vi "Variant To String.vi"(4 "Type Enum [auto]":T1, 5 "Formatting (auto)":string, 6 "Variant Type\\default":variant, 7 "Name (error)":string, 8 "error in (no error)":errorcluster, 10 "Multiply":variant, 11 "Registry Object":refnum<class "Carya Config.lvclass">) -> (0 "error out":errorcluster, 2 "String":string, 3 "Registry Object":refnum<class "Carya Config.lvclass">)   [LabVIEW 2013, in "Carya Config.lvclass"]
doc: "Copyright 2018, Carya Automatisering, Wiebe Walstra."
uses:
  Carya Config.lvclass
  <vilib>/Utility/VariantDataType/Type.ctl
  <vilib>/Utility/error.llb/Error Cluster From Error Code.vi
  <vilib>/regexp/Match Regular Expression.xnode
  <vilib>/ErrorRing/Error Ring.xnode
  <vilib>/Utility/VariantDataType/VariantType.lvlib
  CConfig Variant Accessor/CConfig Variant Accessor.lvclass
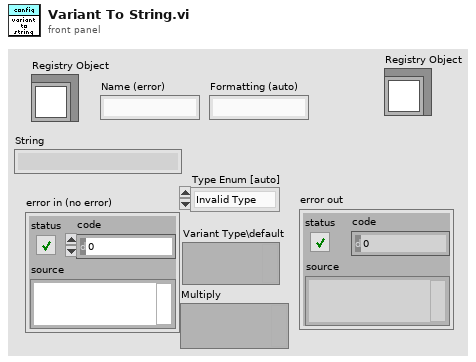
[diagram p1: front panel]
types:
  T1 = typedef "VariantType.lvlib/Type.ctl" = enum8{"Invalid Type", "Void", "I8", "I16", "I32", "I64", "U8", "U16", "U32", "U64", "Single Float", "Double Float", "Extended Float", "Single Complex", "Double Complex", "Extended Complex", "Enum U8", "Enum U16", "Enum U32", "Enum U64", "Single Float With Unit", "Double Float With Unit", "Extended Float With Unit", "Single Complex with Unit", "Double Complex with Unit", "Extended Complex with Unit", "Boolean", "String", "Path", "Picture", "Tag", "Array", "Cluster", "Variant", "LV Variant", "Waveform", "Timestamp", "Digital Waveform", "Digital Data", "ExpressData", "Refnum", "External Data", "VI", "Poly VI", "LabVIEW Class Instance", "Fixed Point"}
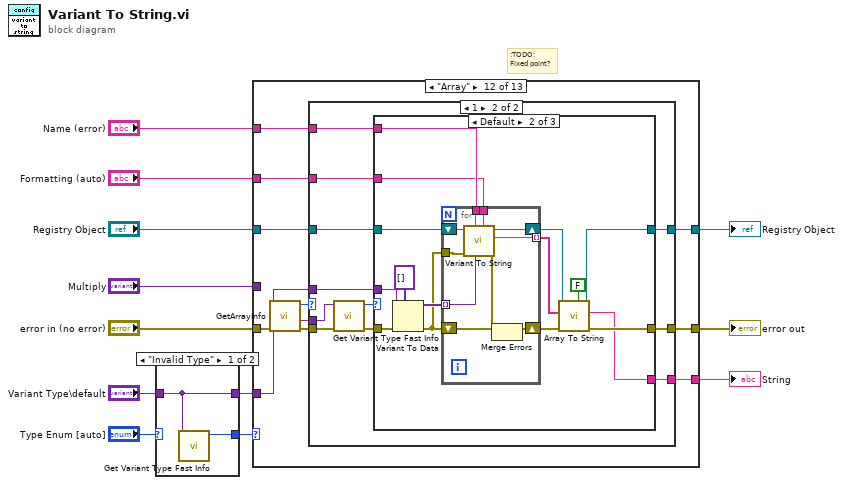
[diagram p0: block diagram]
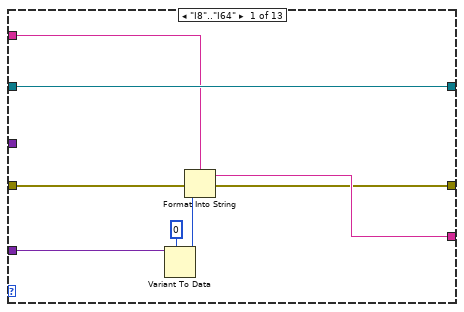
[diagram p2: hidden frame]
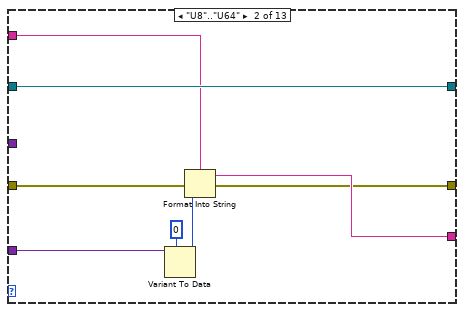
[diagram p3: hidden frame]
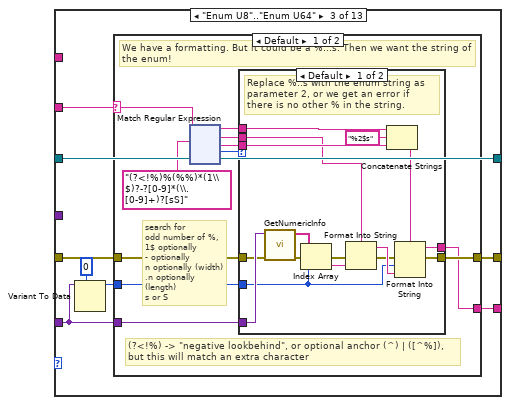
[diagram p4: hidden frame]
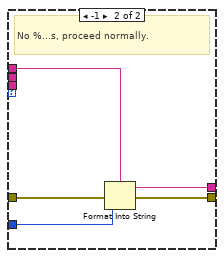
[diagram p5: hidden frame]
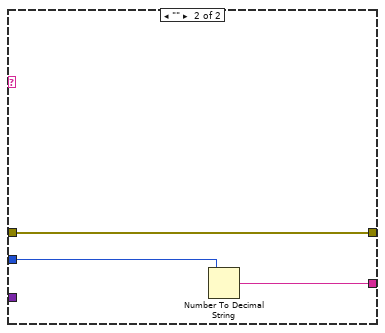
[diagram p6: hidden frame]
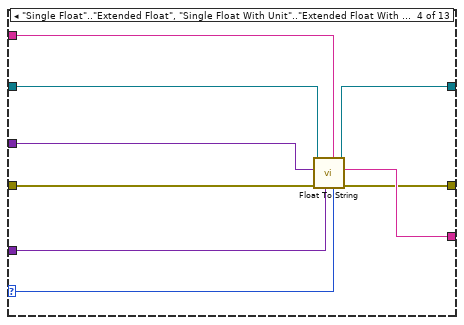
[diagram p7: hidden frame]
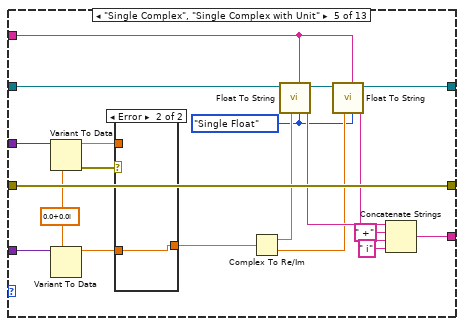
[diagram p8: hidden frame]
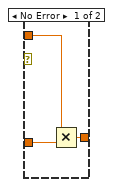
[diagram p9: hidden frame]
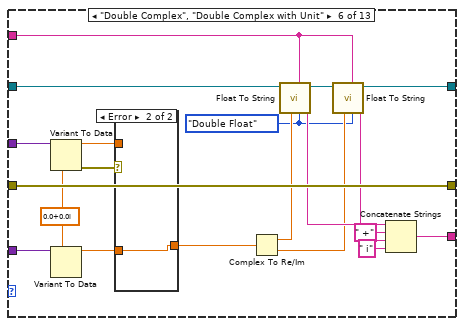
[diagram p10: hidden frame]
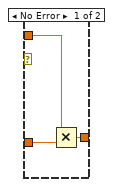
[diagram p11: hidden frame]
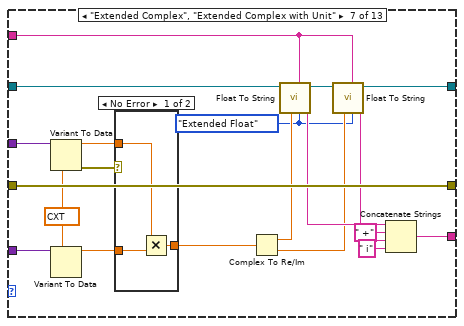
[diagram p12: hidden frame]
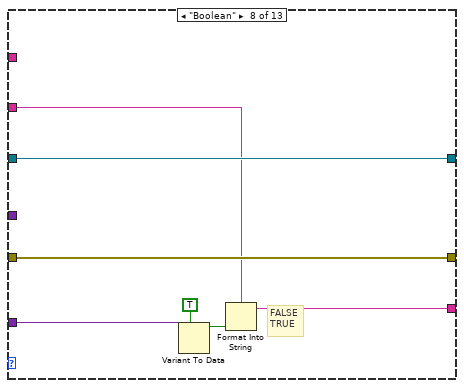
[diagram p14: hidden frame]
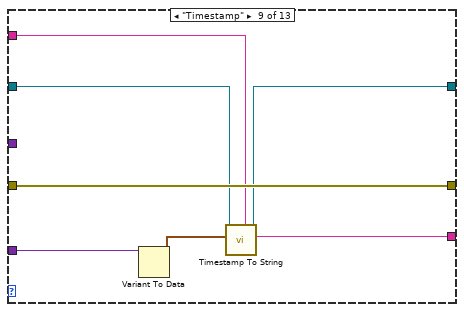
[diagram p15: hidden frame]
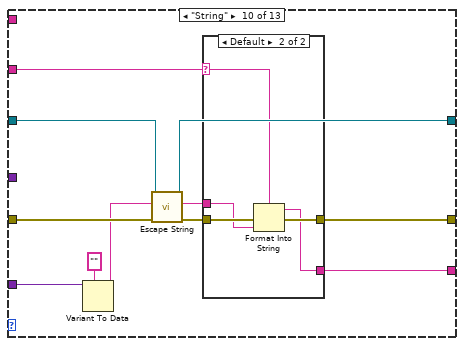
[diagram p16: hidden frame]
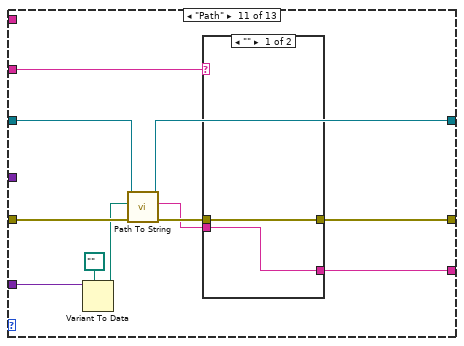
[diagram p18: hidden frame]
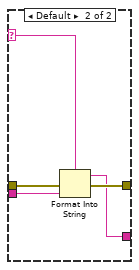
[diagram p19: hidden frame]
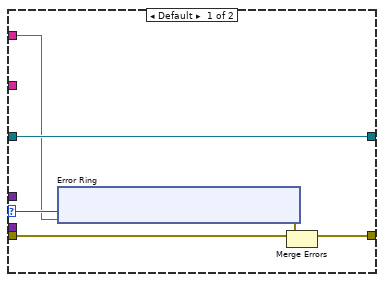
[diagram p20: hidden frame]
diagram:
  # ":TODO:\nFixed point?"
  n1 = case shown="\"Invalid Type\"" "Type Enum [auto]" {
    selector: "Type Enum [auto]" -> [_ w16]
    tunnel: "Variant Type\\default" -> [w13 w15]
    tunnel: [w14 w16] -> w7
    tunnel: [w13 w15] -> w8
    frame "Invalid Type" {
      n2 = call "Get Variant Type Fast Info.vi"("Variant"=w13) -> ("Type Enum"=w14:T1)  [unwired: 6 in, 4 out]
    }
    frame Default {
    }
  }
  n3 = case shown="\"Array\"" w7 {
    selector: w7 -> [_ _ _ w190 _ _ _ _ _ _ _ _ w409]
    tunnel: [w17 w25 w36 w191 w217 w241 w265 w274 w282 w287 w306 w328 w411] -> w10
    tunnel: "error in (no error)" -> [w18 w26 w37 w193 w217 w241 w265 w274 w282 w293 w311 w322 w413]
    tunnel: "Registry Object" -> [w20 w29 w40 w194 w204 w228 w252 w273 w281 w291 w309 w330 w412]
    tunnel: [w20 w29 w40 w197 w215 w239 w263 w273 w280 w290 w308 w329 w412] -> w4
    tunnel: w8 -> [w24 w32 w34 w192 w206 w230 w254 w276 w283 w294 w312 w327 _]
    tunnel: [w21 w28 w39 w196 w210 w234 w258 w271 w277 w285 w304 w325 _] -> w6
    tunnel: "Name (error)" -> [_ _ _ _ _ _ _ _ _ _ _ w324 w406]
    tunnel: "Formatting (auto)" -> [w19 w27 w38 w195 w209 w233 w257 w270 w278 w284 w303 w320 _]
    tunnel: "Multiply" -> [_ _ _ w189 w203 w227 w251 _ _ _ _ _ _]
    frame "I8".."I64" {
      n4 = Variant To Data(type=i64 0, Variant=w24) -> (data=w22:i64)  [unwired: 1 in, 1 out]
      n5 = Format Into String(format string=w19, error in=w18, w22) -> (resulting string=w21:string, error out=w17:errorcluster)  [unwired: 1 in]
    }
    frame "U8".."U64" {
      n6 = Variant To Data(type=u64 0, Variant=w32) -> (data=w30:u64)  [unwired: 1 in, 1 out]
      n7 = Format Into String(format string=w27, error in=w26, w30) -> (resulting string=w28:string, error out=w25:errorcluster)  [unwired: 1 in]
    }
    frame "Enum U8".."Enum U64" {
      n8 = Variant To Data(type=u64 0 ("unsigned 64bit integer"), Variant=w34) -> (data=w33:u64)  [unwired: 1 in, 1 out]
      n9 = case shown="Default" w38 {
        selector: w38 -> [w46 _]
        tunnel: w34 -> [w45 _]
        tunnel: [w42 w188] -> w39
        tunnel: w37 -> [w44 w186]
        tunnel: [w43 w186] -> w36
        tunnel: w33 -> [w41 w187]
        frame Default {
          # "(?<!%) -> \"negative lookbehind\", or optional anchor (^) | ([^%]), but this will match an extra character"
          # "search for\nodd number of %,\n1$ optionally\n- optionally\nn optionally (width)\n.n optionally (length)\ns or S"
          # "We have a formatting. But it could be a %...s. Then we want the string of the enum!"
          n10 = xnode "Match Regular Expression"("input string"=w46, "regular expression"="(?<!%)%(%%)*(1\\$)?-?[0-9]*(\\.[0-9]+)?[sS]") -> ("before match"=w49:string, "whole match"=w50:string, "after match"=w51:string, "offset past match"=w48:i32)  [unwired: 4 in, 1 out]
          n11 = case shown="Default" w48 {
            tunnel: w49 -> [w66 w68]
            tunnel: [w62 w67] -> w42
            tunnel: w50 -> [w52 _]
            tunnel: w45 -> [w59 _]
            tunnel: w51 -> [w63 _]
            tunnel: w44 -> [w58 w71]
            tunnel: [w55 w70] -> w43
            tunnel: w41 -> [w54 w69]
            frame Default {
              # "Replace %..s with the enum string as parameter 2, or we get an error if there is no other % in the string."
              n12 = call <vilib>:"GetNumericInfo.vi"("error in (no error)"=w58, "Variant"=w59) -> ("error out"=w57:errorcluster, "EnumNames"=w65:string[])  [unwired: 6 in, 2 out]
              n13 = Index Array(array=w65, index=w54) -> (element=w64:string)
              n14 = Format Into String(format string=w52, error in=w57, w64) -> (resulting string=w61:string, error out=w56:errorcluster)  [unwired: 1 in]
              n15 = Concatenate Strings(w66, "%2$s" ("string"), w63) -> (w53:string)
              n16 = Format Into String(format string=w53, error in=w56, w54, w61) -> (resulting string=w62:string, error out=w55:errorcluster)  [unwired: 1 in]
            }
            frame -1 {
              # "No %...s, proceed normally."
              n17 = Format Into String(format string=w68, error in=w71, w69) -> (resulting string=w67:string, error out=w70:errorcluster)  [unwired: 1 in]
            }
          }
        }
        frame "" {
          n18 = Number To Decimal String(number=w187) -> (decimal integer string=w188:string)  [unwired: 1 in]
        }
      }
    }
    frame "Single Float".."Extended Float", "Single Float With Unit".."Extended Float With Unit" {
      n19 = call-dynamic "Float To String.vi"("Type Enum [auto]"=w190, "Formatting (auto)"=w195, "Variant"=w192, "error in (no error)"=w193, "Multiply"=w189, "Registry Object"=w194) -> ("error out"=w191:errorcluster, "resulting string"=w196:string, "Registry Object"=w197:refnum<class "Carya Config.lvclass">)  [unwired: 3 in]
    }
    frame "Single Complex", "Single Complex with Unit" {
      w205 = Type."Single Float" ("Type Enum [auto]")
      w198 = csg 0.0+0.0i
      n20 = Variant To Data(type=w198, Variant=w203) -> (data=w200:csg, error out=w199:errorcluster)  [unwired: 1 in]
      n21 = Variant To Data(type=w198, Variant=w206) -> (data=w202:csg)  [unwired: 1 in, 1 out]
      n22 = case shown="Error" w199 {
        tunnel: w202 -> [w220 w221]
        tunnel: [w219 w221] -> w201
        tunnel: w200 -> [w218 _]
        frame No Error {
          n23 = Multiply(x=w218, y=w220) -> (x*y=w219:csg)
        }
        frame Error {
        }
      }
      n24 = Complex To Re/Im(x + iy=w201) -> (x=w208:sgl, y=w207:sgl)
      n25 = call-dynamic "Float To String.vi"("Type Enum [auto]"=w205, "Formatting (auto)"=w209, "Variant"=w208, "Registry Object"=w204) -> ("resulting string"=w214:string, "Registry Object"=w216:refnum<class "Carya Config.lvclass">)  [unwired: 5 in, 1 out]
      n26 = call-dynamic "Float To String.vi"("Type Enum [auto]"=w205, "Formatting (auto)"=w209, "Variant"=w207, "Registry Object"=w216) -> ("resulting string"=w212:string, "Registry Object"=w215:refnum<class "Carya Config.lvclass">)  [unwired: 5 in, 1 out]
      n27 = Concatenate Strings(w214, " +" ("string"), w212, " i" ("string")) -> (w210:string)
    }
    frame "Double Complex", "Double Complex with Unit" {
      w229 = Type."Double Float" ("Type Enum [auto]")
      w222 = cdb 0.0+0.0i
      n28 = Variant To Data(type=w222, Variant=w227) -> (data=w224:cdb, error out=w223:errorcluster)  [unwired: 1 in]
      n29 = Variant To Data(type=w222, Variant=w230) -> (data=w226:cdb)  [unwired: 1 in, 1 out]
      n30 = case shown="Error" w223 {
        tunnel: w226 -> [w244 w245]
        tunnel: [w243 w245] -> w225
        tunnel: w224 -> [w242 _]
        frame No Error {
          n31 = Multiply(x=w242, y=w244) -> (x*y=w243:cdb)
        }
        frame Error {
        }
      }
      n32 = Complex To Re/Im(x + iy=w225) -> (x=w232:dbl, y=w231:dbl)
      n33 = call-dynamic "Float To String.vi"("Type Enum [auto]"=w229, "Formatting (auto)"=w233, "Variant"=w232, "Registry Object"=w228) -> ("resulting string"=w238:string, "Registry Object"=w240:refnum<class "Carya Config.lvclass">)  [unwired: 5 in, 1 out]
      n34 = call-dynamic "Float To String.vi"("Type Enum [auto]"=w229, "Formatting (auto)"=w233, "Variant"=w231, "Registry Object"=w240) -> ("resulting string"=w236:string, "Registry Object"=w239:refnum<class "Carya Config.lvclass">)  [unwired: 5 in, 1 out]
      n35 = Concatenate Strings(w238, " +" ("string"), w236, " i" ("string")) -> (w234:string)
    }
    frame "Extended Complex", "Extended Complex with Unit" {
      w253 = Type."Extended Float" ("Type Enum [auto]")
      w246 = cxt 0.0+0.0i
      n36 = Variant To Data(type=w246, Variant=w251) -> (data=w248:cxt, error out=w247:errorcluster)  [unwired: 1 in]
      n37 = Variant To Data(type=w246, Variant=w254) -> (data=w250:cxt)  [unwired: 1 in, 1 out]
      n38 = case shown="No Error" w247 {
        tunnel: w250 -> [w268 w269]
        tunnel: [w267 w269] -> w249
        tunnel: w248 -> [w266 _]
        frame No Error {
          n39 = Multiply(x=w266, y=w268) -> (x*y=w267:cxt)
        }
        frame Error {
        }
      }
      n40 = Complex To Re/Im(x + iy=w249) -> (x=w256:ext, y=w255:ext)
      n41 = call-dynamic "Float To String.vi"("Type Enum [auto]"=w253, "Formatting (auto)"=w257, "Variant"=w256, "Registry Object"=w252) -> ("resulting string"=w262:string, "Registry Object"=w264:refnum<class "Carya Config.lvclass">)  [unwired: 5 in, 1 out]
      n42 = call-dynamic "Float To String.vi"("Type Enum [auto]"=w253, "Formatting (auto)"=w257, "Variant"=w255, "Registry Object"=w264) -> ("resulting string"=w260:string, "Registry Object"=w263:refnum<class "Carya Config.lvclass">)  [unwired: 5 in, 1 out]
      n43 = Concatenate Strings(w262, " +" ("string"), w260, " i" ("string")) -> (w258:string)
    }
    frame "Boolean" {
      # "FALSE\nTRUE"
      n44 = Variant To Data(type=TRUE, Variant=w276) -> (data=w272:bool)  [unwired: 1 in, 1 out]
      n45 = Format Into String(format string=w270, w272) -> (resulting string=w271:string)  [unwired: 2 in, 1 out]
    }
    frame "Timestamp" {
      n46 = Variant To Data(Variant=w283) -> (data=w279:timestamp)  [unwired: 2 in, 1 out]
      n47 = call-dynamic "Timestamp To String.vi"("Formatting (auto)"=w278, "Time Stamp"=w279, "Registry Object"=w281) -> ("String"=w277:string, "Registry Object"=w280:refnum<class "Carya Config.lvclass">)  [unwired: 6 in, 1 out]
    }
    frame "String" {
      n48 = Variant To Data(type="" ("regular expression"), Variant=w294) -> (data=w289:string)  [unwired: 1 in, 1 out]
      n49 = call-dynamic "Escape String.vi"("error in (no error)"=w293, "String"=w289, "Registry Object"=w291) -> ("error out"=w288:errorcluster, "Escaped string"=w286:string, "Registry Object"=w290:refnum<class "Carya Config.lvclass">)  [unwired: 6 in]
      n50 = case shown="Default" w284 {
        selector: w284 -> [_ w297]
        tunnel: w288 -> [w296 w301]
        tunnel: [w296 w300] -> w287
        tunnel: w286 -> [w295 w299]
        tunnel: [w295 w298] -> w285
        frame "" {
        }
        frame Default {
          n51 = Format Into String(format string=w297, error in=w301, w299) -> (resulting string=w298:string, error out=w300:errorcluster)  [unwired: 1 in]
        }
      }
    }
    frame "Path" {
      n52 = Variant To Data(type=path "" ("regular expression"), Variant=w312) -> (data=w302:path)  [unwired: 1 in, 1 out]
      n53 = call-dynamic "Path To String.vi"("error in (no error)"=w311, "Path"=w302, "Registry Object"=w309) -> ("error out"=w307:errorcluster, "resulting string"=w305:string, "Registry Object"=w308:refnum<class "Carya Config.lvclass">)  [unwired: 6 in]
      n54 = case shown="\"\"" w303 {
        selector: w303 -> [_ w315]
        tunnel: w307 -> [w313 w319]
        tunnel: [w313 w318] -> w306
        tunnel: w305 -> [w314 w317]
        tunnel: [w314 w316] -> w304
        frame "" {
        }
        frame Default {
          n55 = Format Into String(format string=w315, error in=w319, w317) -> (resulting string=w316:string, error out=w318:errorcluster)  [unwired: 1 in]
        }
      }
    }
    frame "Array" {
      n56 = call <vilib>:"GetArrayInfo.vi"("error in (no error)"=w322, "Variant"=w327) -> ("error out"=w321:errorcluster, "ArrayElement"=w323:variant, "NDims"=w326:i32)  [unwired: 6 in, 1 out]
      n57 = case shown="1" w326 {
        selector: w326 -> [w335 _]
        tunnel: w330 -> [w336 w353]
        tunnel: [w336 w352] -> w329
        tunnel: [w334 w354] -> w328
        tunnel: w327 -> [_ w350]
        tunnel: [_ w355] -> w325
        tunnel: w324 -> [w332 w351]
        tunnel: w323 -> [_ w349]
        tunnel: w321 -> [w331 w348]
        tunnel: w320 -> [_ w345]
        frame Default {
          n58 = xnode "Error Ring"("parameter 0"=w335, "parameter 1"=w332) -> ("error out"=w333:errorcluster)
          n59 = Merge Errors(w331, w333) -> (w334:errorcluster)
        }
        frame 1 {
          n60 = call "Get Variant Type Fast Info.vi"("error in (no error)"=w348, "Variant"=w349) -> ("error out"=w347:errorcluster, "Type Enum"=w346:T1)  [unwired: 5 in, 3 out]
          n61 = case shown="Default" w346 {
            tunnel: [_ w370 w396] -> w355
            tunnel: [w357 w374 w398] -> w354
            tunnel: w353 -> [w360 w379 w393]
            tunnel: [w360 w372 w397] -> w352
            tunnel: w351 -> [w356 w378 _]
            tunnel: w350 -> [_ w377 w400]
            tunnel: w347 -> [w359 w375 w399]
            tunnel: w345 -> [_ w369 _]
            frame "Cluster" {
              n62 = xnode "Error Ring"("parameter 0"=w356) -> ("error out"=w358:errorcluster)
              n63 = Merge Errors(w359, w358) -> (w357:errorcluster)
            }
            frame Default {
              n64 = Variant To Data(error in=w375, type=variant[] [], Variant=w377) -> (data=w381:variant[], error out=w376:errorcluster)
              n65 = for {
                tunnel: w381 -> [w392] mode=indexing
                shift-right: [w388] -> w380
                shift-left: w376 -> [w390]
                shift-right: [w386] -> w373
                shift-left: w379 -> [w387]
                tunnel: w376 -> [w391]
                tunnel: [w385] -> w371 mode=indexing
                tunnel: w378 -> [w384]
                tunnel: w369 -> [w383]
                n66 = call-dynamic "Variant To String.vi"("Formatting (auto)"=w383, "Variant Type\\default"=w392, "Name (error)"=w384, "error in (no error)"=w391, "Registry Object"=w387) -> ("error out"=w389:errorcluster, "String"=w385:string, "Registry Object"=w386:refnum<class "Carya Config.lvclass">)  [unwired: 4 in]
                n67 = Merge Errors(w390, w389) -> (w388:errorcluster)
              }
              n68 = call-dynamic "Array To String.vi"("Escape string? [T]"=FALSE, "error in (no error)"=w380, "Array"=w371, "Registry Object"=w373) -> ("error out"=w374:errorcluster, "resulting string"=w370:string, "Registry Object"=w372:refnum<class "Carya Config.lvclass">)  [unwired: 5 in]
            }
            frame "String" {
              n69 = Variant To Data(error in=w399, type=string[] [], Variant=w400) -> (data=w395:string[], error out=w394:errorcluster)
              n70 = call-dynamic "Array To String.vi"("error in (no error)"=w394, "Array"=w395, "Registry Object"=w393) -> ("error out"=w398:errorcluster, "resulting string"=w396:string, "Registry Object"=w397:refnum<class "Carya Config.lvclass">)  [unwired: 6 in]
            }
          }
        }
      }
    }
    frame Default {
      n71 = Format Into String(w409) -> (resulting string=w408:string)  [unwired: 3 in, 1 out]
      n72 = Concatenate Strings(" (" ("string"), w406, ")" ("string")) -> (w403:string)
      n73 = Empty String/Path?(string/path=w406) -> (empty?=w407:bool)
      n74 = Select(t=w406, s=w407, f=w403) -> (s? t:f=w402:string)
      n75 = xnode "Error Ring"("parameter 0"=w408, "parameter 1"=w402) -> ("error out"=w410:errorcluster)
      n76 = Merge Errors(w413, w410) -> (w411:errorcluster)
    }
  }
  "Registry Object" <- w4
  "error out" <- w10
  "String" <- w6
